vi "RANSAC.vi"(9 "Checks":dbl, 10 "XY Array":T1[](array[typedef]), 11 "Tolerance":dbl) -> (2 "Best Line":cluster{"M":dbl, "B":dbl, "Strength":dbl})   [LabVIEW 2016]
uses:
  040-typeDefs/LidarPoint.ctl
  <vilib>/Analysis/NI_AALPro.lvlib
panel:
  in  "Line":cluster{"M":dbl, "B":dbl, "Strength":dbl}
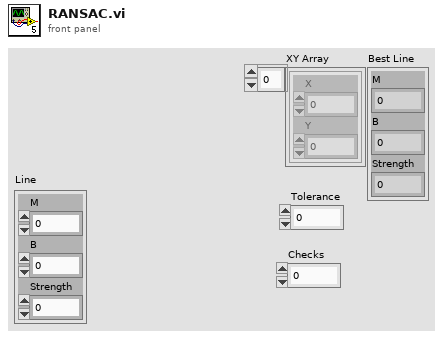
[diagram p1: front panel]
types:
  T1 = typedef "LidarPoint.ctl" = cluster{"X":dbl, "Y":dbl}
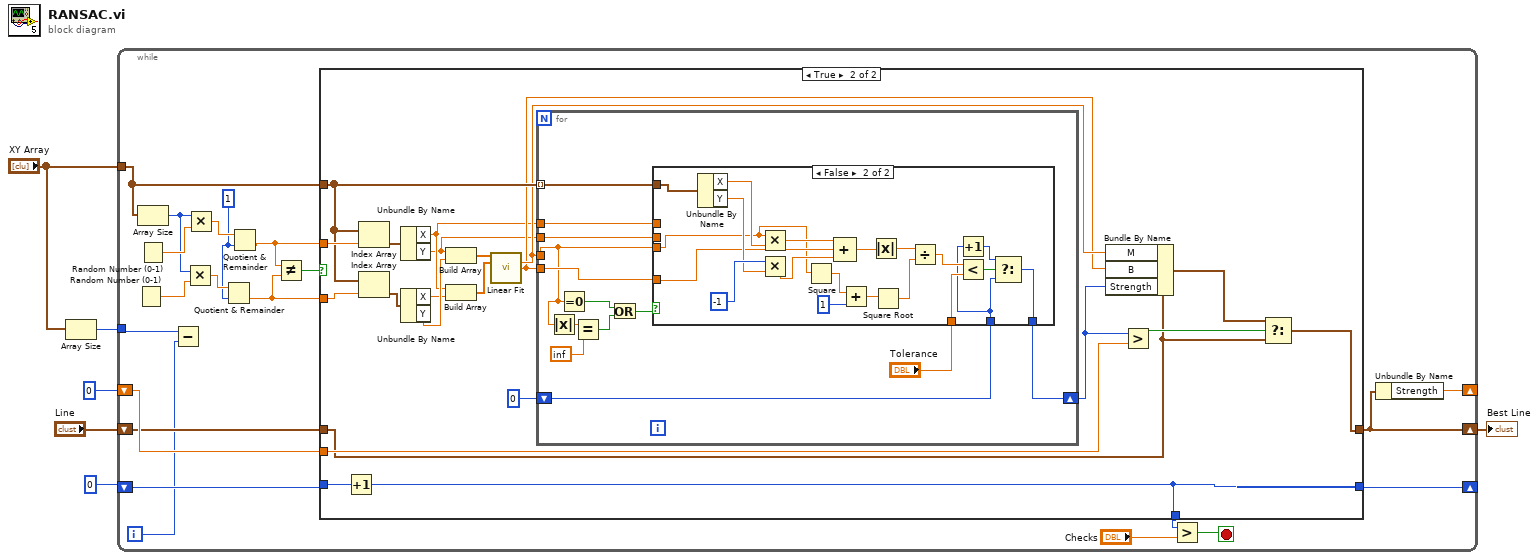
[diagram p0: block diagram]
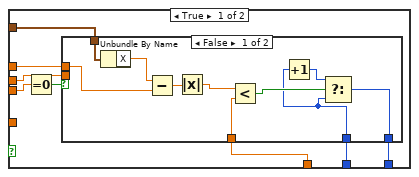
[diagram p3: hidden frame]
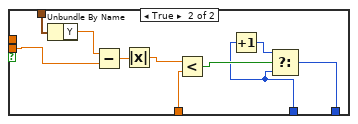
[diagram p4: hidden frame]
diagram:
  n1 = Array Size(array="XY Array") -> (size(s)=w1:i32)
  n2 = while {
    tunnel: "XY Array" -> [w19]
    shift-right: [w20] -> _
    shift-left: 0 -> [w23]
    shift-right: [w14] -> _
    shift-left: 0 -> [w17]
    shift-right: [w15] -> w3
    shift-left: "Line" -> [w16]
    tunnel: w1 -> [w10]
    i -> [w9]
    stop <- w22 stop-if-true
    w11 = 1
    n3 = Random Number (0-1)() -> (number: 0 to 1=w26:dbl)
    n4 = Array Size(array=w19) -> (size(s)=w25:i32)
    n5 = Random Number (0-1)() -> (number: 0 to 1=w27:dbl)
    n6 = Subtract(x=w10, y=w9) -> ()  [unwired: 1 out]
    n7 = Multiply(x=w25, y=w26) -> (x*y=w12:dbl)
    n8 = Multiply(x=w25, y=w27) -> (x*y=w13:dbl)
    n9 = Quotient & Remainder(x=w12, y=w11) -> (floor(x/y)=w7:dbl)  [unwired: 1 out]
    n10 = Quotient & Remainder(x=w13, y=w11) -> (floor(x/y)=w8:dbl)  [unwired: 1 out]
    n11 = Not Equal?(x=w8, y=w7) -> (x != y?=w24:bool)
    n12 = case shown="True" w24 {
      tunnel: w23 -> [w29 w51]
      tunnel: [w29 w50] -> w21
      tunnel: [w29 w50] -> w20
      tunnel: w19 -> [_ w41]
      tunnel: w8 -> [_ w49]
      tunnel: w7 -> [_ w48]
      tunnel: w17 -> [_ w38]
      tunnel: w16 -> [w28 w32]
      tunnel: [w28 w34] -> w15
      frame False {
      }
      frame True {
        n13 = Increment(x=w51) -> (x+1=w50:i32)
        n14 = Index Array(array=w41, index=w49) -> (element=w47:T1)
        n15 = Index Array(array=w41, index=w48) -> (element=w46:T1)
        n16 = Unbundle By Name(w47) -> ("X"=w31:dbl, "Y"=w30:dbl)
        n17 = Unbundle By Name(w46) -> ("X"=w44:dbl, "Y"=w45:dbl)
        n18 = Build Array(w30, w45) -> (w43:dbl[])
        n19 = Build Array(w31, w44) -> (w42:dbl[])
        n20 = call <vilib>:"Linear Fit.vi"("Y"=w43, "X"=w42) -> ("slope"=w37:dbl, "intercept"=w36:dbl)  [unwired: 9 in, 3 out]
        n21 = for {
          tunnel: w37 -> [w56]
          tunnel: w36 -> [w64]
          tunnel: w41 -> [w63] mode=indexing
          shift-right: [w60] -> w35
          shift-left: 0 -> [w61]
          tunnel: w31 -> [w59]
          tunnel: w30 -> [w58]
          n22 = Absolute Value(x=w56) -> (abs(x)=w57:dbl)
          n23 = Equal To 0?(x=w56) -> (x = 0?=w53:bool)
          n24 = Equal?(x=w57, y=inf) -> (x = y?=w52:bool)
          n25 = Or(x=w53, y=w52) -> (x .or. y?=w54:bool)
          n26 = case shown="False" w54 {
            tunnel: w64 -> [_ w107]
            tunnel: w63 -> [w70 w112]
            tunnel: "Tolerance" -> [w68 w97]
            tunnel: w61 -> [w67 w95]
            tunnel: [w66 w94] -> w60
            tunnel: w59 -> [w69 _]
            tunnel: w58 -> [w65 _]
            tunnel: w56 -> [w71 w93]
            frame True {
              n27 = Equal To 0?(x=w71) -> (x = 0?=w72:bool)
              n28 = case shown="False" w72 {
                tunnel: w70 -> [w82 w92]
                tunnel: w69 -> [w80 _]
                tunnel: w68 -> [w78 w89]
                tunnel: w67 -> [w74 w85]
                tunnel: [w73 w84] -> w66
                tunnel: w65 -> [_ w83]
                frame False {
                  n29 = Unbundle By Name(w82) -> ("X"=w81:dbl)
                  n30 = Subtract(x=w81, y=w80) -> (x-y=w79:dbl)
                  n31 = Absolute Value(x=w79) -> (abs(x)=w77:dbl)
                  n32 = Less?(x=w77, y=w78) -> (x < y?=w76:bool)
                  n33 = Increment(x=w74) -> (x+1=w75:i32)
                  n34 = Select(t=w75, s=w76, f=w74) -> (s? t:f=w73:i32)
                }
                frame True {
                  n35 = Unbundle By Name(w92) -> ("Y"=w91:dbl)
                  n36 = Subtract(x=w91, y=w83) -> (x-y=w90:dbl)
                  n37 = Absolute Value(x=w90) -> (abs(x)=w88:dbl)
                  n38 = Less?(x=w88, y=w89) -> (x < y?=w87:bool)
                  n39 = Increment(x=w85) -> (x+1=w86:i32)
                  n40 = Select(t=w86, s=w87, f=w85) -> (s? t:f=w84:i32)
                }
              }
            }
            frame False {
              n41 = Unbundle By Name(w112) -> ("X"=w109:dbl, "Y"=w110:dbl)
              n42 = Multiply(x=w93, y=w109) -> (x*y=w108:dbl)
              n43 = Multiply(x=-1, y=w110) -> (x*y=w106:dbl)
              n44 = Square(x=w93) -> (x^2=w103:dbl)
              n45 = Compound Arithmetic op=ADD(w108, w107, w106) -> (w105:dbl)
              n46 = Add(x=w103, y=1) -> (x+y=w101:dbl)
              n47 = Absolute Value(x=w105) -> (abs(x)=w104:dbl)
              n48 = Square Root(x=w101) -> (sqrt(x)=w100:dbl)
              n49 = Divide(x=w104, y=w100) -> (x/y=w99:dbl)
              n50 = Increment(x=w95) -> (x+1=w96:i32)
              n51 = Less?(x=w99, y=w97) -> (x < y?=w98:bool)
              n52 = Select(t=w96, s=w98, f=w95) -> (s? t:f=w94:i32)
            }
          }
        }
        n53 = Bundle By Name(cluster=w32, "M"=w37, "B"=w36, "Strength"=w35) -> (w33:cluster{"M":dbl, "B":dbl, "Strength":dbl})
        n54 = Greater?(x=w35, y=w38) -> (0:w39:bool)
        n55 = Select(t=w33, s=w39, f=w32) -> (s? t:f=w34:cluster{"M":dbl, "B":dbl, "Strength":dbl})
      }
    }
    n56 = Greater?(x=w21, y="Checks") -> (0:w22:bool)
    n57 = Unbundle By Name(w15) -> ("Strength"=w14:dbl)
  }
  "Best Line" <- w3
